vi "tra.vi"(9 "t2":dbl format="%#_13g", 10 "dt(s)":dbl, 11 "i":i32) -> (0 "complet?":bool, 1 "t2?":bool, 2 "Waveform Chart":dbl(graph), 3 "second":dbl, 4 "t3":dbl)   [LabVIEW 2019]
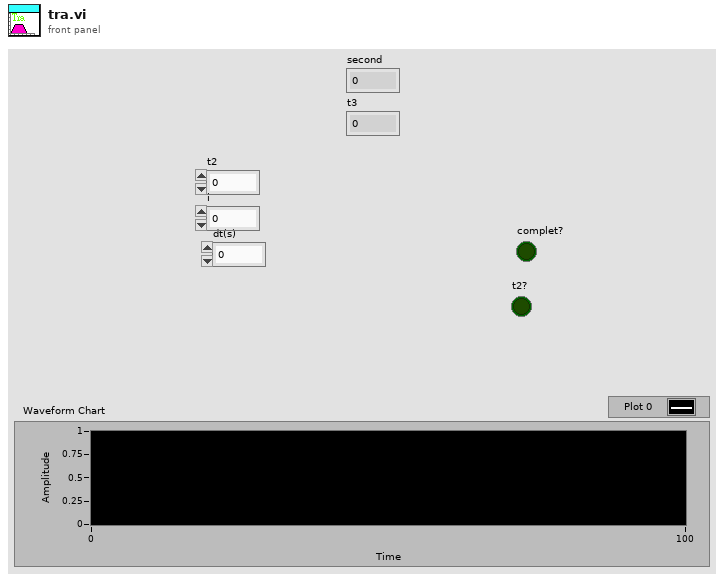
[diagram p1: front panel]
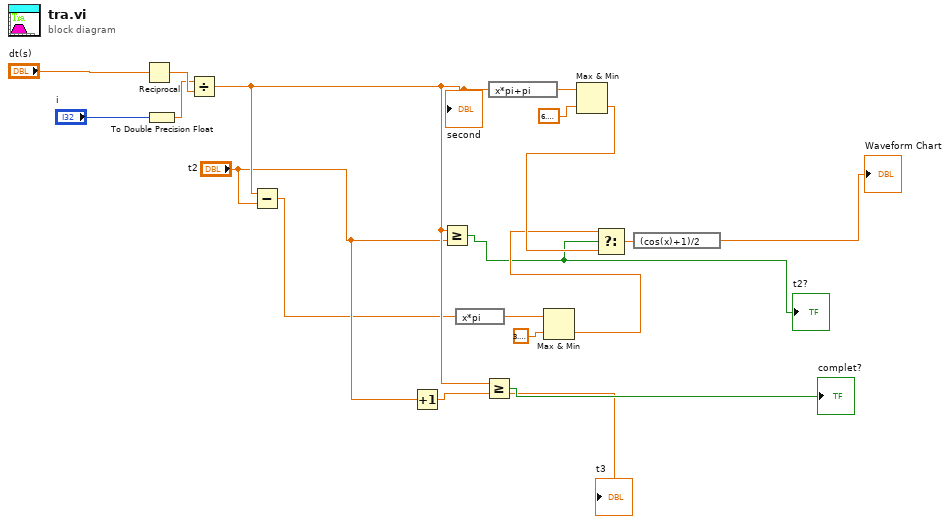
[diagram p0: block diagram]
diagram:
  n1 = Reciprocal(x="dt(s)") -> (1/x=w13:dbl)
  n2 = To Double Precision Float(number="i") -> (double precision float=w5:dbl)
  n3 = Divide(x=w5, y=w13) -> (x/y=w3:dbl)
  "second" <- w3
  n4 = Subtract(x=w3, y="t2") -> (x-y=w1:dbl)
  n5 = Increment(x="t2") -> (x+1=w7:dbl)
  "t3" <- w7
  n6 = Greater Or Equal?(x=w3, y="t2") -> (x >= y?=w6:bool)
  "t2?" <- w6
  n7 = expression code="x*pi"(w1) -> (w12:dbl)
  n8 = Greater Or Equal?(x=w3, y=w7) -> (x >= y?=→"complet?":bool)
  n9 = expression code="x*pi+pi"(w3) -> (w17:dbl)
  n10 = Max & Min(x=w12, y=3.141592653589793) -> (min(x,y)=w10:dbl)  [unwired: 1 out]
  n11 = Max & Min(x=w17, y=6.283185307179586) -> (min(x,y)=w15:dbl)  [unwired: 1 out]
  n12 = Select(t=w10, s=w6, f=w15) -> (s? t:f=w14:dbl)
  n13 = expression code="(cos(x)+1)/2"(w14) -> (→"Waveform Chart":dbl)
